vi "Start Async.vi"(8 "error in (no error)":errorcluster, 11 "gRPC Server in":refnum<class "Greeter.lvclass">) -> (0 "error out":errorcluster, 3 "gRPC Server out":refnum<class "Greeter.lvclass">)   [LabVIEW 2019, in "Generated_server.lvlib" / "Greeter.lvclass"]
uses:
  Greeter.lvclass
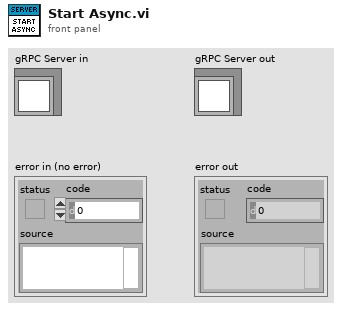
[diagram p1: front panel]
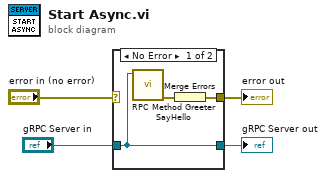
[diagram p0: block diagram]
diagram:
  n1 = case shown="No Error" "error in (no error)" {
    selector: "error in (no error)" -> [_ w9]
    tunnel: [w7 w9] -> w3
    tunnel: [w6 w8] -> w1
    tunnel: "gRPC Server in" -> [w6 w8]
    frame No Error {
      n2 = call "RPC Method Greeter SayHello.vi"("OOP Server in"=w6) -> ("error out"=w5:errorcluster)  [unwired: 9 in, 1 out]
      n3 = Merge Errors(w5) -> (w7:errorcluster)
    }
    frame Error {
    }
  }
  "error out" <- w3
  "gRPC Server out" <- w1
